vi "DAQ_spectrum_analyzer_simultaneous_averaged_diag.vi"(0 "Samples per Channel":i32=100000, 1 "minimum value":dbl=-1.0, 2 "DC voltage (V)":dbl, 3 "maximum value":dbl=1.0, 4 "LD channel":tag="Dev3/ai0", 5 "Error In":errorcluster, 6 "Rate":dbl=5000.0, 7 "Ref channel":tag="Dev3/ai2", 8 "Second":bool) -> (9 "Unbalanced?":bool, 10 "Starting Time of DAQ":dbl, 11 "raw signal waveform":waveform(dbl), 12 "MLD Timetrace":waveform(dbl)={"t0"=timestamp(0 s since 1904-01-01), "dt"=0.005, "Y"=array[4000 elements]}, 13 "2f Frequency":dbl[](array[numeric])=[6.0], 14 "Calculated frequency":dbl=6.0, 15 "Reference Timetrace":waveform(dbl)={"t0"=timestamp(0 s since 1904-01-01), "dt"=0.0002, "Y"=array[100000 elements]}, 16 "1f 2f":T1, 17 "FFT - (mVRMS/DC)":cluster{"f0":dbl, "df":dbl, "magnitude":dbl[]}, 18 "2f Peak Amplitude (mVrms/V)":dbl=0.004981012167818904, 19 "error out":errorcluster)   [LabVIEW 2013]
uses:
  <vilib>/DAQmx/read.llb/DAQmx Read (Analog 2D DBL NChan NSamp).vi
  <vilib>/Analysis/baseanly.llb/Mean (DBL).vi
  <vilib>/DAQmx/create/channels.llb/DAQmx Create Channel (AI-Voltage-Basic).vi
  <vilib>/DAQmx/configure/timing.llb/DAQmx Timing (Sample Clock).vi
  <vilib>/DAQmx/miscellaneous.llb/DAQmx Fill In Error Info.vi
  <vilib>/express/express analysis/Spectral/Block/exnSpectralBlock spectral measurements RMS poly.vi
  <vilib>/express/express analysis/Spectral/Block/exnSpectralBlock spectral measurements RMS WFM.vi
  <vilib>/express/express analysis/Spectral/XNode/ExpressSpectralMeasurementsBlockNode.xnode
  <resource>/objmgr/daqmx.rc
  <vilib>/Analysis/NI_AALBase.lvlib
panel:
  out "Original":waveform(dbl)[](graph)
  out "Triggered":waveform(dbl)[](graph)
  out "1f Frequency":dbl[](array[numeric])
  out "1f Peak Amplitude(mVrms/V)":dbl
  out "t0":dbl
  out "raw":dbl[](array[numeric])
  out "Rising edges":i32=120
  in  "Peak FWHM":dbl=0.1
  out "Waveform Graph 3":cluster{"f0":dbl, "df":dbl, "magnitude":dbl[]}[](graph)=[{"f0"=0.0, "df"=0.05, "magnitude"=array[50000 elements]}, {"f0"=0.0, "df"=0.05, "magnitude"=array[2000 elements]}]
  out "Waveform Graph 2":waveform(dbl)(graph)={"t0"=timestamp(0 s since 1904-01-01), "dt"=0.0002, "Y"=array[100000 elements]}
  out "Waveform Graph":waveform(dbl)(graph)={"t0"=timestamp(0 s since 1904-01-01), "dt"=0.005, "Y"=array[4000 elements]}
  out "Spectra":cluster{"f0":dbl, "df":dbl, "magnitude":dbl[]}[](array[cluster])=[{"f0"=0.0, "df"=0.05, "magnitude"=array[50000 elements]}, {"f0"=0.0, "df"=0.05, "magnitude"=array[2000 elements]}]
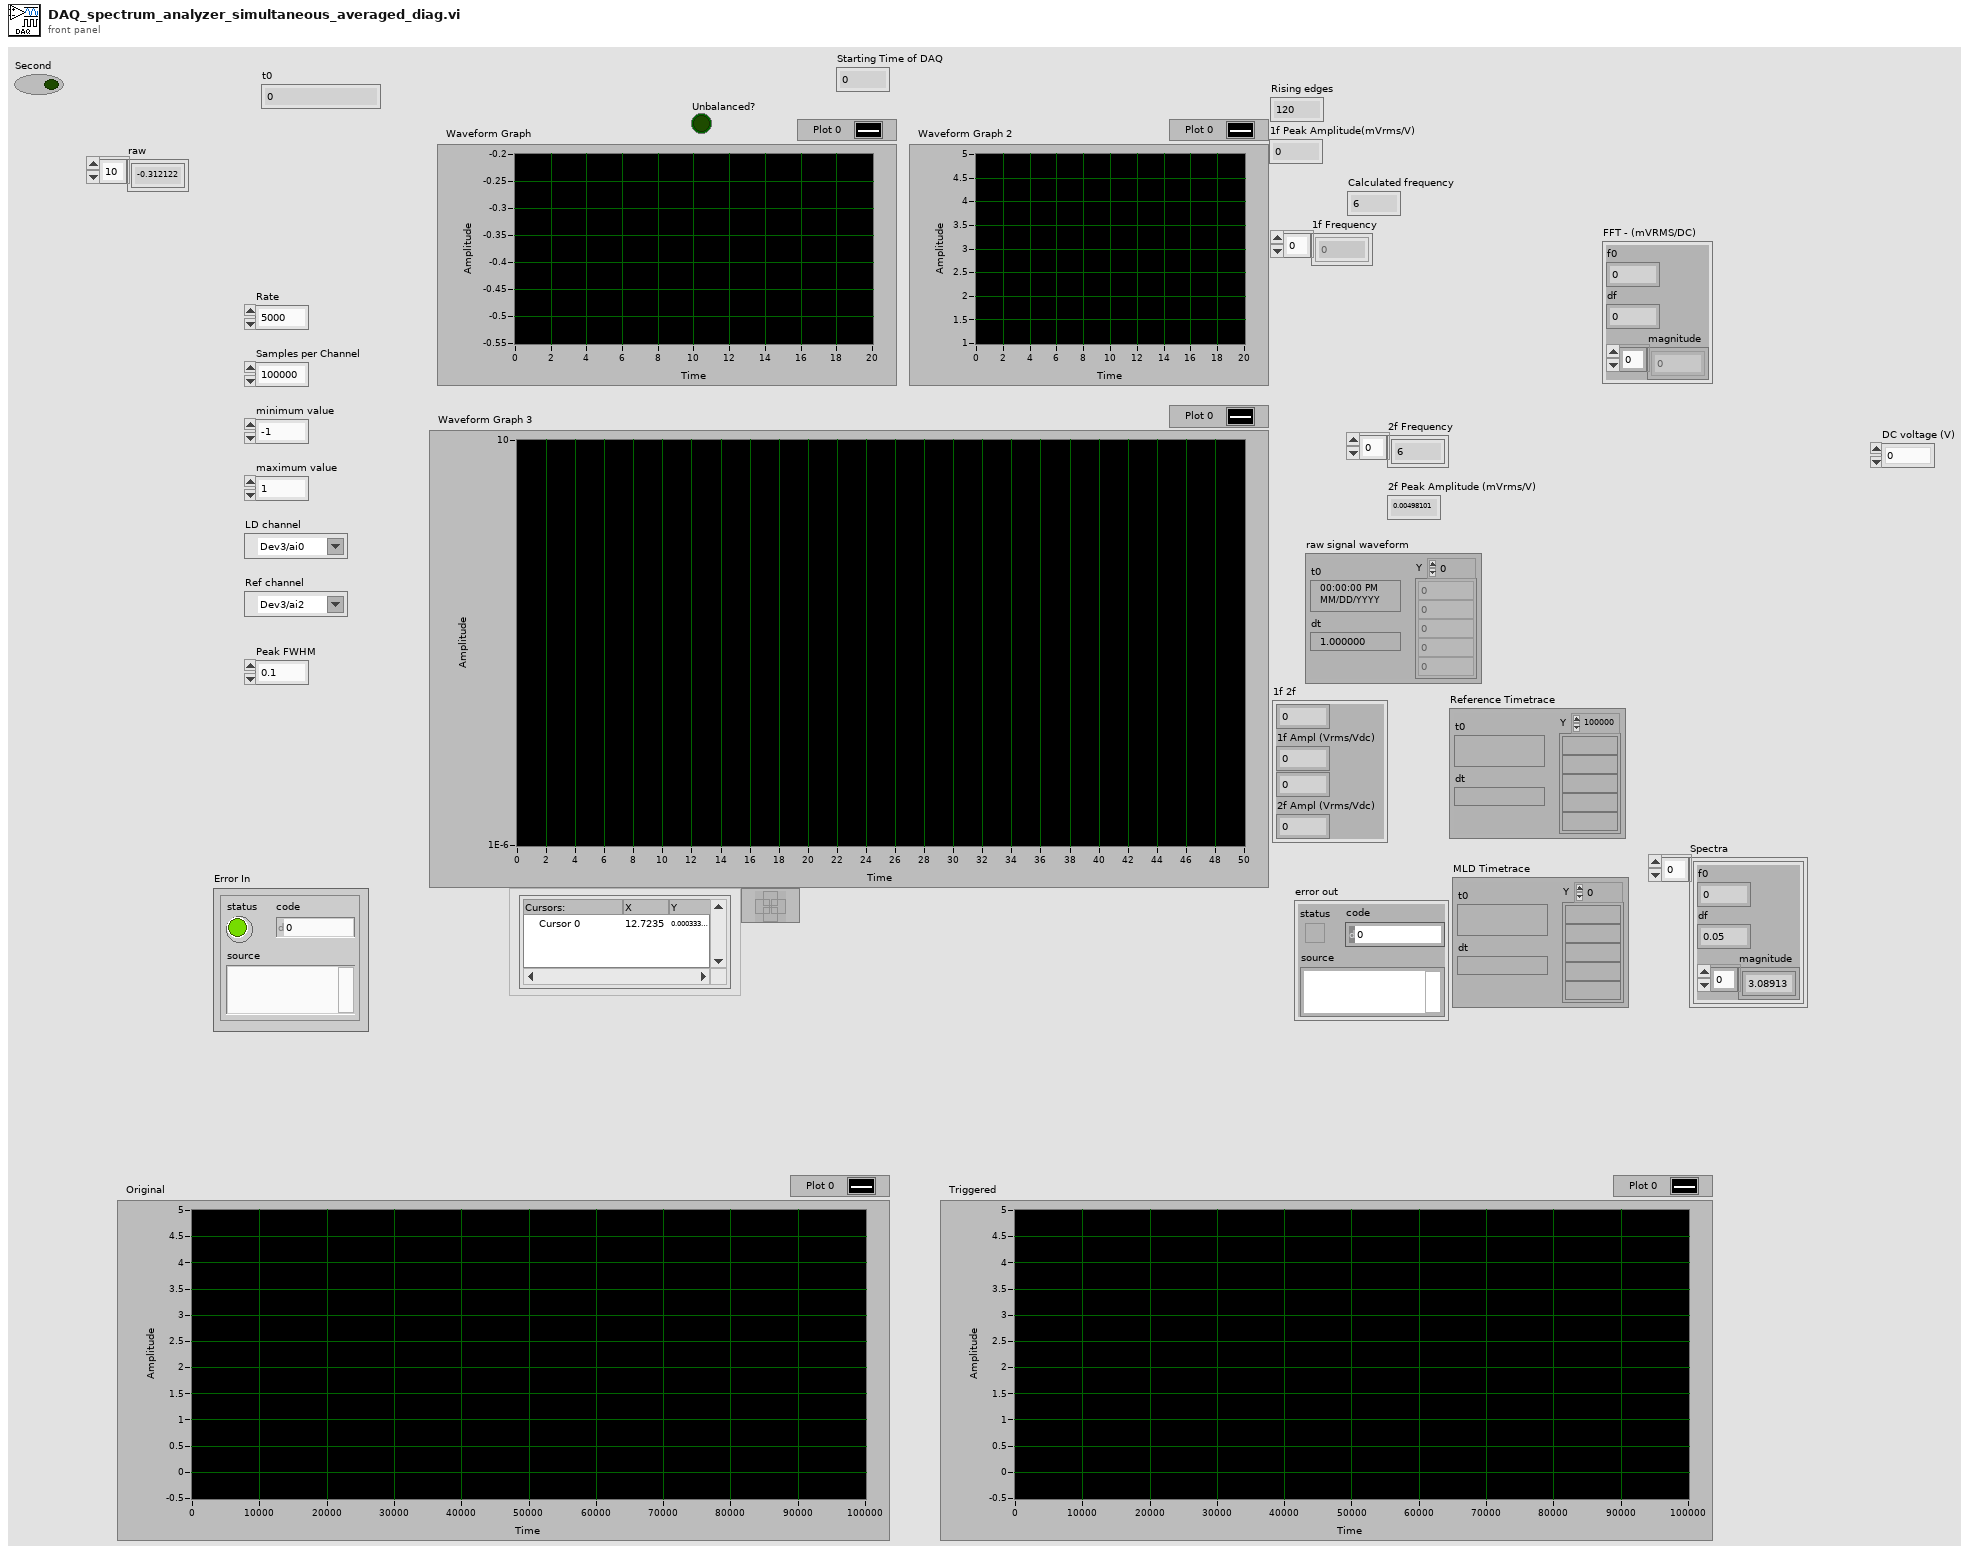
[diagram p1: front panel]
types:
  T1 = cluster{dbl, "1f Ampl (Vrms/Vdc)":dbl, dbl, "2f Ampl (Vrms/Vdc)":dbl}
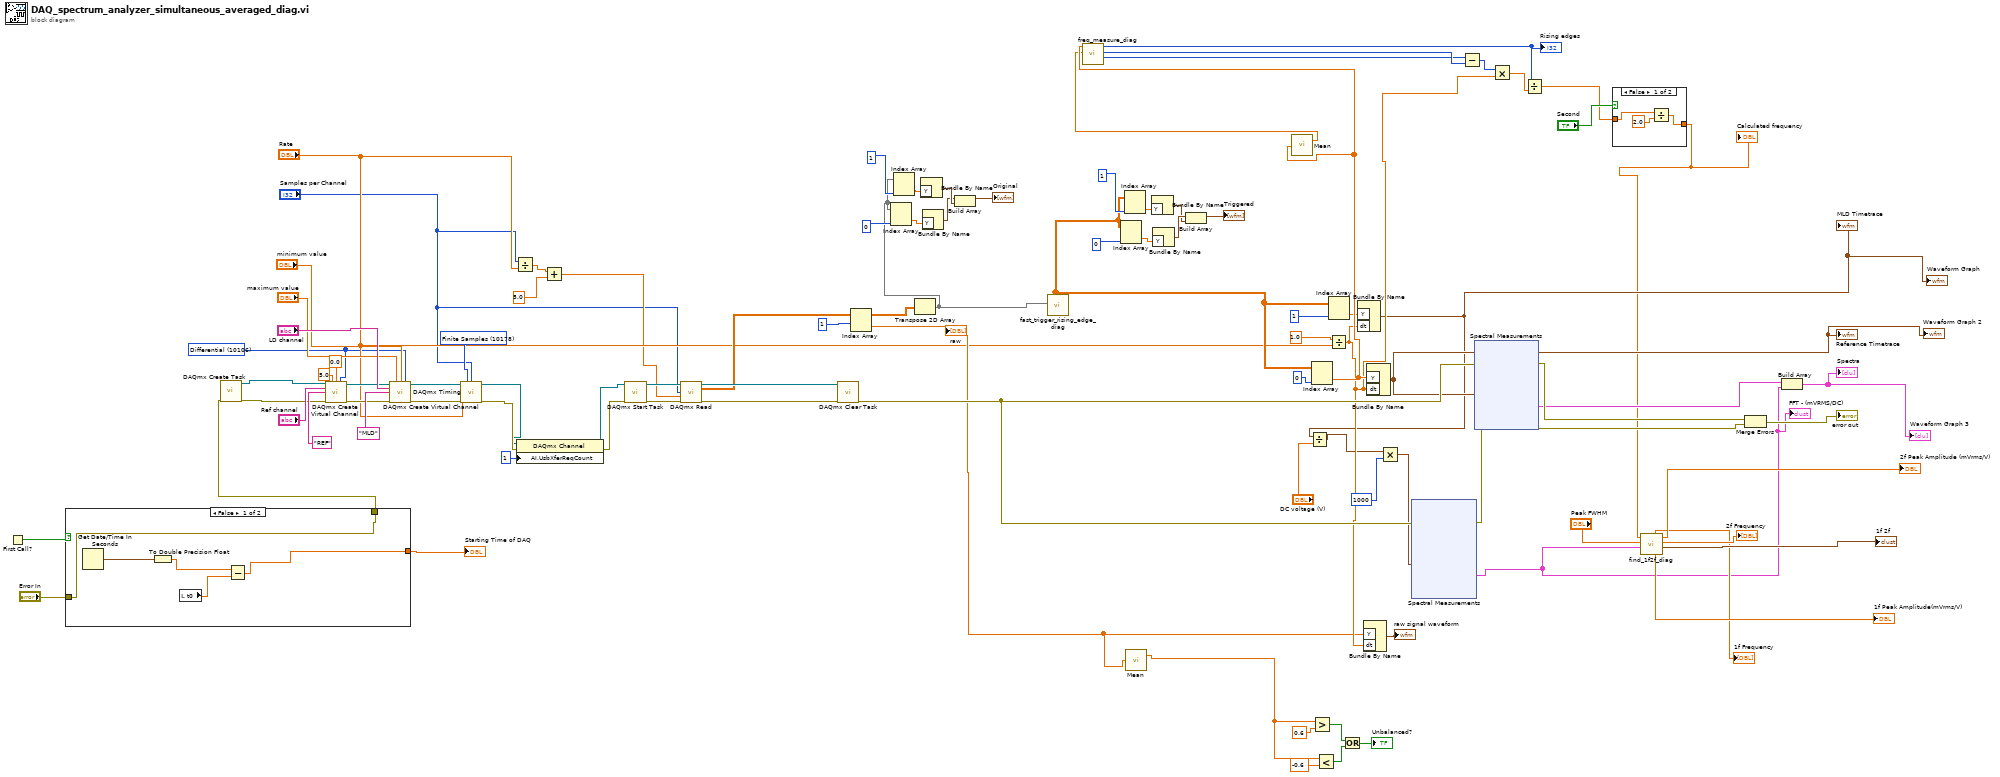
[diagram p0: block diagram]
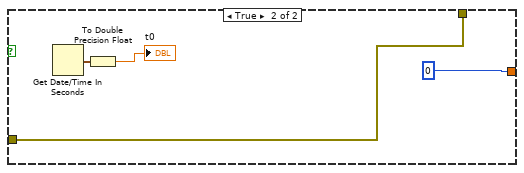
[diagram p3: hidden frame]
diagram:
  w1 = 10106 items=["default"=-1, "RSE"=10083, "NRSE"=10078, "Differential"=10106, "Pseudodifferential"=12529] ("input terminal configuration")
  w83 = 10178 items=["Finite Samples"=10178, "Continuous Samples"=10123] ("sample mode")
  n1 = First Call?() -> (First Call?: T/F=w67:bool)
  n2 = case shown="False" w67 {
    tunnel: [w96 0] -> w66
    tunnel: [w95 w100] -> w25
    tunnel: "Error In" -> [w95 w100]
    frame False {
      n3 = Get Date/Time In Seconds() -> (seconds since 1Jan1904=w97:timestamp)
      n4 = To Double Precision Float(number=w97) -> (double precision float=w98:dbl)
      n5 = local read "t0"() -> (w99:dbl)
      n6 = Subtract(x=w98, y=w99) -> (x-y=w96:dbl)
    }
    frame True {
      n7 = Get Date/Time In Seconds() -> (seconds since 1Jan1904=w103:timestamp)
      n8 = To Double Precision Float(number=w103) -> (double precision float=→"t0":dbl)
    }
  }
  "Starting Time of DAQ" <- w66
  n9 = call <vilib>:"DAQmx Create Task.vi"("error in"=w25) -> ("task out"=w26:refnum<k21>, "error out"=w24:errorcluster)  [unwired: 13 in]
  n10 = call-poly <vilib>:"DAQmx Create Virtual Channel.vi"("task in"=w26, "maximum value"=5.0, "minimum value"=0.0, "input terminal configuration"=w1, "physical channels"="Ref channel", "name to assign"="REF", "error in"=w24) -> ("task out"=w72:refnum<k21>, "error out"=w77:errorcluster)  [unwired: 7 in]
  n11 = call-poly <vilib>:"DAQmx Create Virtual Channel.vi"("task in"=w72, "maximum value"="maximum value", "minimum value"="minimum value", "input terminal configuration"=w1, "physical channels"="LD channel", "name to assign"="MLD", "error in"=w77) -> ("task out"=w88:refnum<k21>, "error out"=w89:errorcluster)  [unwired: 7 in]
  n12 = call-poly <vilib>:"DAQmx Timing.vi"("task/channels in"=w88, "sample mode"=w83, "samples per channel"="Samples per Channel", "rate"="Rate", "error in"=w89) -> ("task out"=w20:refnum<k21>, "error out"=w22:errorcluster)  [unwired: 9 in]
  n13 = Divide(x="Samples per Channel", y="Rate") -> (x/y=w30:dbl)
  n14 = property class="DAQmx Channel"(reference=w20, error in=w22, "AI.UsbXferReqCount"=u32 1) -> (reference out=w19:refnum<k21>, error out=w21:errorcluster)
  n15 = Add(x=w30, y=5.0) -> (x+y=w28:dbl)
  n16 = call <vilib>:"DAQmx Start Task.vi"("task/channels in"=w19, "error in"=w21) -> ("task out"=w85:refnum<k21>, "error out"=w86:errorcluster)  [unwired: 12 in]
  n17 = call-poly <vilib>:"DAQmx Read.vi"("task/channels in"=w85, "number of samples per channel"="Samples per Channel", "timeout"=w28, "error in"=w86) -> ("task out"=w84:refnum<k21>, "data"=w39:dbl[][], "error out"=w82:errorcluster)  [unwired: 9 in]
  n18 = call <vilib>:"DAQmx Clear Task.vi"("task in"=w84, "error in"=w82) -> ("error out"=w92:errorcluster)  [unwired: 13 in]
  n19 = Index Array(array=w39, index (row)=1) -> (element=w33:dbl[])  [unwired: 1 in]
  "raw" <- w33
  n20 = Transpose 2D Array(2D array=w39) -> (transposed array=w5:dbl[][])
  n21 = Index Array(array=w5, index (col)=0 ("disabled index (col)")) -> (element=w7:dbl[])  [unwired: 1 in]
  n22 = Index Array(array=w5, index (col)=1 ("disabled index (col)")) -> (element=w8:dbl[])  [unwired: 1 in]
  n23 = Bundle By Name("Y"=w8) -> (w12:waveform(dbl))  [unwired: 1 in]
  n24 = Bundle By Name("Y"=w7) -> (w11:waveform(dbl))  [unwired: 1 in]
  n25 = Build Array(w11, w12) -> (→"Original":waveform(dbl)[])
  n26 = call "fast_trigger_rising_edge_diag.vi"("Ref_MLD measurement"=w5) -> ("Ref_MLD_triggered"=w37:dbl[][])  [unwired: 7 in, 3 out]
  n27 = Index Array(array=w37, index (col)=0 ("disabled index (col)")) -> (element=w45:dbl[])  [unwired: 1 in]
  n28 = Index Array(array=w37, index (col)=1 ("disabled index (col)")) -> (element=w44:dbl[])  [unwired: 1 in]
  n29 = call-poly <vilib>:"Mean.vi"("X"=w33) -> ("mean"=w32:dbl)  [unwired: 1 out]
  n30 = Bundle By Name("Y"=w44) -> (w35:waveform(dbl))  [unwired: 1 in]
  n31 = Bundle By Name("Y"=w45) -> (w36:waveform(dbl))  [unwired: 1 in]
  n32 = Build Array(w36, w35) -> (→"Triggered":waveform(dbl)[])
  n33 = Index Array(array=w37, index (col)=0 ("index (row)")) -> (element=w64:dbl[])  [unwired: 1 in]
  n34 = call-poly <vilib>:"Mean.vi"("X"=w64) -> ("mean"=w63:dbl)  [unwired: 1 out]
  n35 = call "freq_measure_diag.vi"("Ref_average"=w63, "data"=w64) -> ("Actual (last) Rising edge index"=w55:i32, "First Rising edge index"=w56:i32, "Rising edges"=w52:i32)  [unwired: 7 in]
  "Rising edges" <- w52
  n36 = Greater?(x=w32, y=0.6) -> (0:w48:bool)
  n37 = Less?(x=w32, y=-0.6) -> (x < y?=w49:bool)
  n38 = Index Array(array=w37, index (col)=1 ("index (row)")) -> (element=w38:dbl[])  [unwired: 1 in]
  n39 = Divide(x=1.0, y="Rate") -> (x/y=w41:dbl)
  n40 = Or(x=w48, y=w49) -> (x .or. y?=→"Unbalanced?":bool)
  n41 = Bundle By Name("Y"=w38, "dt"=w41) -> (w14:waveform(dbl))  [unwired: 1 in]
  "MLD Timetrace" <- w14
  "Waveform Graph" <- w14
  n42 = Divide(x=w14, y="DC voltage (V)") -> (x/y=w16:waveform(dbl))
  n43 = Bundle By Name("Y"=w33, "dt"=w41) -> (→"raw signal waveform":waveform(dbl))  [unwired: 1 in]
  n44 = Bundle By Name("Y"=w64, "dt"=w41) -> (w69:waveform(dbl))  [unwired: 1 in]
  "Reference Timetrace" <- w69
  "Waveform Graph 2" <- w69
  n45 = Multiply(x=w16, y=1000) -> (x*y=w13:waveform(dbl))
  n46 = xnode "Spectral Measurements"("Signals"=w13, "error in (no error)"=w92) -> ("FFT - (RMS)"=w15:cluster{"f0":dbl, "df":dbl, "magnitude":dbl[]}, "error out"=w94:errorcluster)  [unwired: 1 out]
  "FFT - (mVRMS/DC)" <- w15
  n47 = Subtract(x=w55, y=w56) -> (x-y=w54:i32)
  n48 = xnode "Spectral Measurements"("Signals"=w69, "error in (no error)"=w92) -> ("FFT - (RMS)"=w91:cluster{"f0":dbl, "df":dbl, "magnitude":dbl[]}, "error out"=w93:errorcluster)  [unwired: 1 out]
  n49 = Multiply(x=w54, y=w41) -> (x*y=w53:dbl)
  n50 = Divide(x=w52, y=w53) -> (x/y=w3:dbl)
  n51 = case shown="False" "Second" {
    tunnel: [w105 w107] -> w2
    tunnel: w3 -> [w104 w107]
    frame False {
      n52 = Divide(x=w104, y=2.0) -> (x/y=w105:dbl)
    }
    frame True {
    }
  }
  "Calculated frequency" <- w2
  n53 = call "find_1f2f_diag.vi"("FFT - (RMS)"=w15, "Peak FWHM"="Peak FWHM", "Central Frequency"=w2) -> ("Cluster"=→"1f 2f":cluster{dbl, dbl, dbl, dbl}, "2f Frequency"=→"2f Frequency":dbl[], "2f Peak Amplitude (mVrms/Vdc)"=→"2f Peak Amplitude (mVrms/V)":dbl, "1f Peak Amplitude(mVrms/Vdc)"=→"1f Peak Amplitude(mVrms/V)":dbl, "1f Frequency"=→"1f Frequency":dbl[])  [unwired: 4 in]
  n54 = Merge Errors(w93, w94) -> (→"error out":errorcluster)
  n55 = Build Array(w91, w15) -> (→"Spectra" →"Waveform Graph 3":cluster{"f0":dbl, "df":dbl, "magnitude":dbl[]}[])
